vi "1D Fit Insert Fixed Parameters.vi"(6 "Fit Model":T2, 8 "Error In":errorcluster, 9 "Fixed Parameter Names":T1[](array[typedef]), 10 "Fixed Parameter Values":dbl[](array[numeric]), 11 "Fitted Parameters":dbl[](array[numeric])) -> (0 "Error Out":errorcluster, 3 "All Parameters":dbl[](array[numeric]))   [LabVIEW 2021, in "Fits.lvlib"]
uses:
  Fits.lvlib
  Decay Convolution/Decay Model.ctl
  IRF(X)PSED/Decay Fit Parameters In List.ctl
  <vilib>/Utility/error.llb/Error Cluster From Error Code.vi
  <vilib>/ErrorRing/Error Ring.xnode
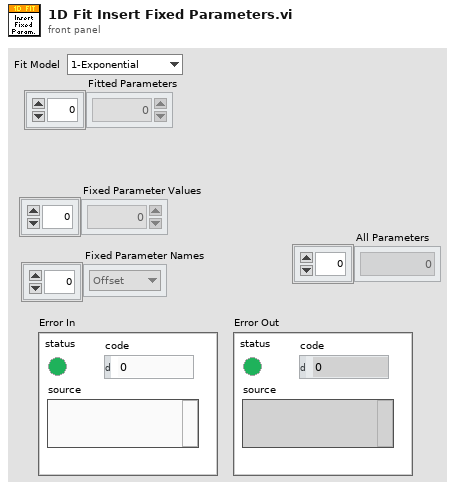
[diagram p1: front panel]
types:
  T1 = typedef "Fits.lvlib/Decay Fit Parameters In List.ctl" = enum16{"Offset", "Baseline", "A_1", "tau_1", "A_2", "tau_2"}
  T2 = typedef "Fits.lvlib/Decay Model.ctl" = enum16{"1-Exponential", "2-Exponentials"}
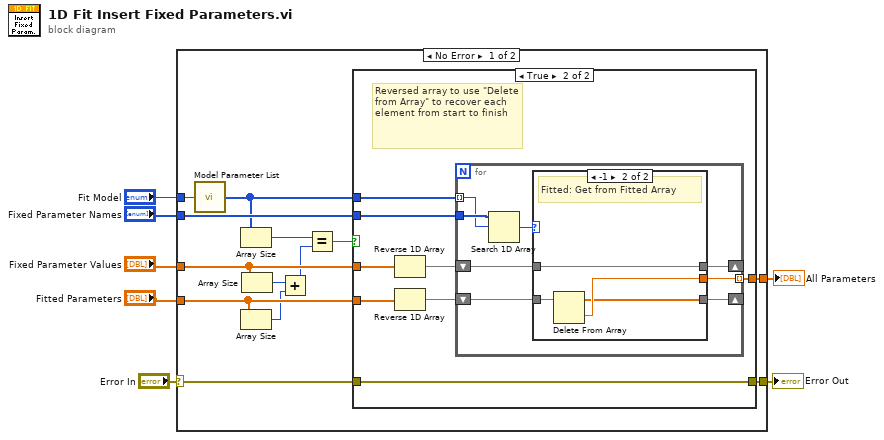
[diagram p0: block diagram]
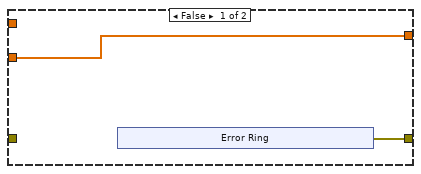
[diagram p2: hidden frame]
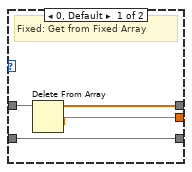
[diagram p3: hidden frame]
diagram:
  n1 = case shown="No Error" "Error In" {
    selector: "Error In" -> [w9 w51]
    tunnel: [w20 _] -> w7
    tunnel: "Fit Model" -> [w19 _]
    tunnel: "Fixed Parameter Names" -> [w18 _]
    tunnel: "Fixed Parameter Values" -> [w16 _]
    tunnel: "Fitted Parameters" -> [w15 _]
    tunnel: [w8 w51] -> w1
    frame No Error {
      n2 = call "Model Parameter List.vi"("Fit Model"=w19) -> ("Model Parameter List"=w17:T1[])
      n3 = Array Size(array=w17) -> (size(s)=w12:i32)
      n4 = Array Size(array=w15) -> (size(s)=w14:i32)
      n5 = Array Size(array=w16) -> (size(s)=w13:i32)
      n6 = Add(x=w13, y=w14) -> (x+y=w11:i32)
      n7 = Equal?(x=w12, y=w11) -> (x = y?=w10:bool)
      n8 = case shown="True" w10 {
        tunnel: [w21 w32] -> w20
        tunnel: w18 -> [_ w31]
        tunnel: w17 -> [_ w30]
        tunnel: w16 -> [_ w29]
        tunnel: w15 -> [w21 w28]
        tunnel: w9 -> [_ w27]
        tunnel: [w22 w27] -> w8
        frame False {
          n9 = xnode "Error Ring"() -> ("error out"=w22:errorcluster)
        }
        frame True {
          # "Reversed array to use \"Delete from Array\" to recover each element from start to finish"
          n10 = Reverse 1D Array(array=w29) -> (reversed array=w34:dbl[])
          n11 = Reverse 1D Array(array=w28) -> (reversed array=w33:dbl[])
          n12 = for {
            tunnel: w30 -> [w36] mode=indexing
            tunnel: w31 -> [w42]
            shift-right: [w38] -> _
            shift-left: w34 -> [w40]
            shift-right: [w37] -> _
            shift-left: w33 -> [w39]
            tunnel: [w35] -> w32 mode=indexing
            n13 = Search 1D Array(1D array=w42, element=w36) -> (index of element=w41:i32)  [unwired: 1 in]
            n14 = case shown="-1" w41 {
              tunnel: w40 -> [w46 w47]
              tunnel: w39 -> [w43 w50]
              tunnel: [w45 w47] -> w38
              tunnel: [w44 w49] -> w35
              tunnel: [w43 w48] -> w37
              frame 0, Default {
                # "Fixed: Get from Fixed Array"
                n15 = Delete From Array(array=w46) -> (deleted portion=w44:dbl, array with subset deleted=w45:dbl[])  [unwired: 2 in]
              }
              frame -1 {
                # "Fitted: Get from Fitted Array"
                n16 = Delete From Array(array=w50) -> (deleted portion=w49:dbl, array with subset deleted=w48:dbl[])  [unwired: 2 in]
              }
            }
          }
        }
      }
    }
    frame Error {
    }
  }
  "All Parameters" <- w7
  "Error Out" <- w1
